vi "CCM-Read Connection Table (I32).vi"(0 "Path In":path, 2 "section":string="Connections", 5 "Endpoints":string[](array[string]), 7 "IOChannels":string[](array[string]), 9 "Channel Names":string[](array[string]), 11 "error in (no error)":errorcluster) -> (4 "Path Out":path, 6 "Endpoints (by channel)":string[](array[string]), 10 "Table":T1[](array[typedef]), 15 "error out":errorcluster)   [LabVIEW 2020]
uses:
  Type Defs/CM-Connection.ctl
  <vilib>/Utility/config.llb/Read Key (I32).vi
  <vilib>/Utility/config.llb/NI_LVConfig.lvlib
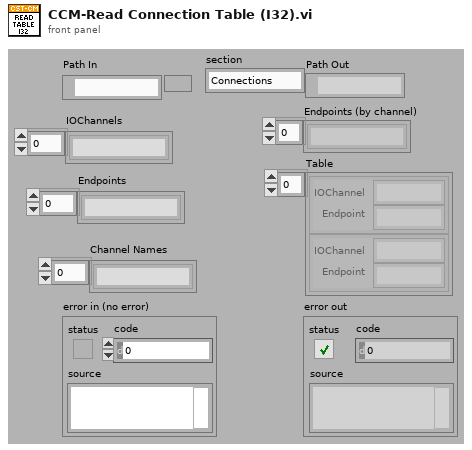
[diagram p1: front panel]
types:
  T1 = typedef "CM-Connection.ctl" = cluster{"IOChannel":string, "Endpoint":string}
  T2 = typedef "NI_LVConfig.lvlib/Config Data RefNum.ctl" = refnum<k1>
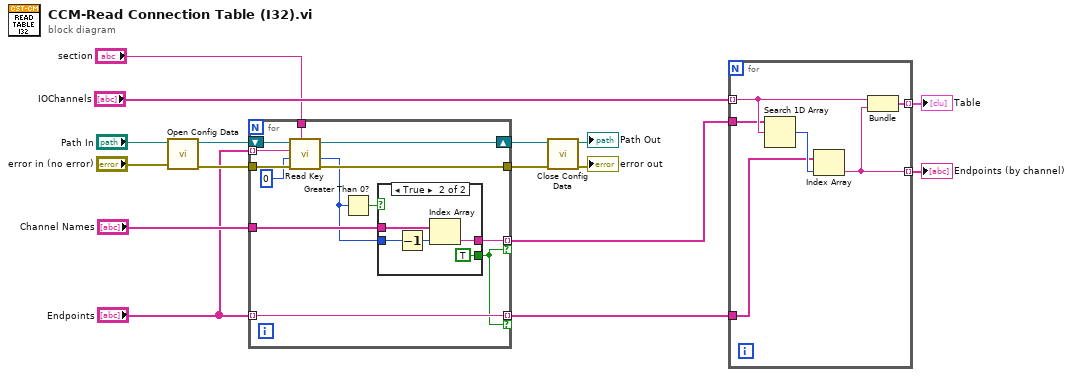
[diagram p0: block diagram]
diagram:
  n1 = call <vilib>:"Open Config Data.vi"("error in (no error)"="error in (no error)", "configuration file path"="Path In") -> ("error out"=w11:errorcluster, "refnum"=w12:T2)  [unwired: 7 in, 1 out]
  n2 = for {
    tunnel: w11 -> [w27]
    tunnel: "Endpoints" -> [w28] mode=indexing
    tunnel: "section" -> [w26]
    tunnel: [w24] -> w9
    shift-right: [w25] -> w10
    shift-left: w12 -> [w29]
    tunnel: "Channel Names" -> [w21]
    tunnel: [w20] -> w3 mode=indexing if=w17
    tunnel: [w18] -> w1 mode=indexing if=w17
    tunnel: "Endpoints" -> [w18] mode=indexing
    n3 = call-poly <vilib>:"Read Key.vi"("section"=w26, "error in (no error)"=w27, "default value"=0, "key"=w28, "refnum"=w29) -> ("error out"=w24:errorcluster, "value"=w19:i32, "refnum out"=w25:T2)  [unwired: 3 in, 1 out]
    n4 = Greater Than 0?(x=w19) -> (x > 0?=w22:bool)
    n5 = case shown="True" w22 {
      tunnel: w21 -> [_ w34]
      tunnel: w19 -> [_ w33]
      tunnel: [_ w32] -> w20
      tunnel: [_ TRUE] -> w17
      frame False {
      }
      frame True {
        n6 = Decrement(x=w33) -> (x-1=w30:i32)
        n7 = Index Array(array=w34, index=w30) -> (element=w32:string)
      }
    }
  }
  n8 = call <vilib>:"Close Config Data.vi"("error in (no error)"=w9, "refnum"=w10) -> ("error out"=→"error out":errorcluster, "file path"=→"Path Out":path)  [unwired: 8 in]
  n9 = for {
    tunnel: "IOChannels" -> [w39] mode=indexing
    tunnel: [w38] -> w8 mode=indexing
    tunnel: [w37] -> w6 mode=indexing
    tunnel: w3 -> [w36]
    tunnel: w1 -> [w35]
    n10 = Search 1D Array(1D array=w36, element=w39) -> (index of element=w40:i32)  [unwired: 1 in]
    n11 = Index Array(array=w35, index=w40) -> (element=w37:string)
    n12 = Bundle("String"=w39, "String"=w37) -> (w38:cluster{"String":string, "String":string})  [unwired: 1 in]
  }
  "Table" <- w8
  "Endpoints (by channel)" <- w6
